vi "Launching Static VI Commit Test.vi"(6 "Open Front Panel?":bool=TRUE, 9 "Data To Set":T1[](array[typedef]), 11 "VI Ref In":refnum<vi>) -> ()   [LabVIEW 2019]
uses:
  TypeDef/Static VI Launch Input.ctl
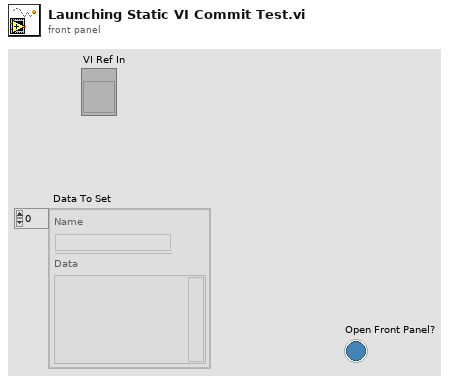
[diagram p1: front panel]
types:
  T1 = typedef "Static VI Launch Input.ctl" = cluster{"Name":string, "Data":variant}
  T2 = enum32{"Bad", "Idle", "Run top level", "Running"}
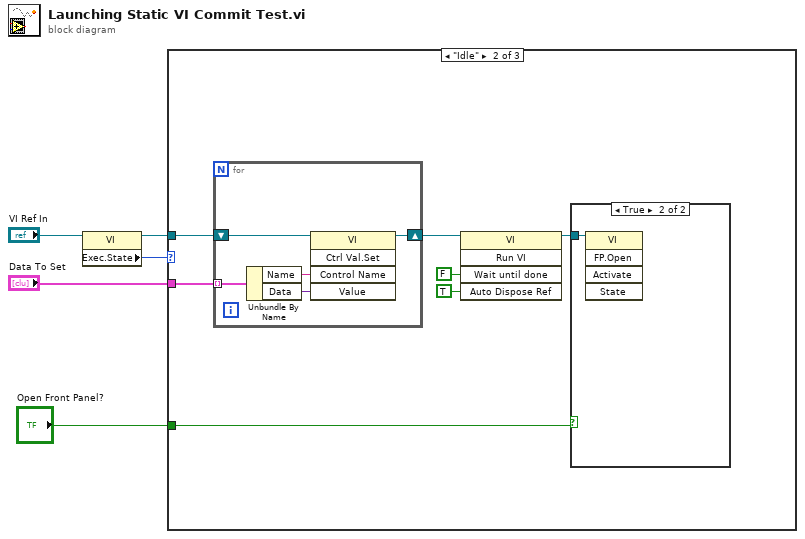
[diagram p0: block diagram]
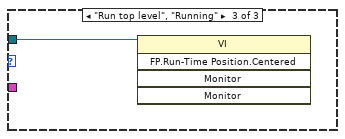
[diagram p4: hidden frame]
diagram:
  n1 = property class="VI"(reference="VI Ref In") -> (reference out=w3:refnum<vi>, "Exec.State"=w4:T2)  [unwired: 1 in, 1 out]
  n2 = case shown="\"Idle\"" w4 {
    tunnel: w3 -> [_ w12 w19]
    tunnel: "Data To Set" -> [_ w11 _]
    tunnel: "Open Front Panel?" -> [_ w6 _]
    frame "Bad", Default {
    }
    frame "Idle" {
      n3 = for {
        tunnel: w11 -> [w17] mode=indexing
        shift-right: [w14] -> w10
        shift-left: w12 -> [w18]
        n4 = Unbundle By Name(w17) -> ("Name"=w16:string, "Data"=w15:variant)
        n5 = invoke class="VI" method="Ctrl Val.Set"(reference=w18, "Control Name"=w16, "Value"=w15) -> (reference out=w14:refnum<vi>)  [unwired: 2 in, 4 out]
      }
      n6 = invoke class="VI" method="Run VI"(reference=w10, "Wait until done"=FALSE ("Wait Until Done"), "Auto Dispose Ref"=TRUE ("Auto Dispose Reference")) -> (reference out=w7:refnum<vi>)  [unwired: 2 in, 4 out]
      n7 = case shown="True" w6 {
        tunnel: w7 -> [_ w13]
        frame False {
        }
        frame True {
          n8 = invoke class="VI" method="FP.Open"(reference=w13) -> ()  [unwired: 4 in, 5 out]
        }
      }
    }
    frame "Run top level", "Running" {
      n9 = invoke class="VI" method="FP.Run-Time Position.Centered"(reference=w19) -> ()  [unwired: 4 in, 5 out]
    }
  }
